vi "Kalman Filter Step.vi"(9 "Control Input":T2, 10 "Observations":T2, 11 "Kalman Filter In":T1) -> (3 "Kalman Filter Out":T1)   [LabVIEW 2020]
uses:
  ctl/Kalman Filter Instance.ctl
  <vilib>/Analysis/Matrix/Datatypes/RealMatrix.ctl
  ctl/Dynamical System Matrices.ctl
  <vilib>/Analysis/Matrix/NI_Matrix.lvlib
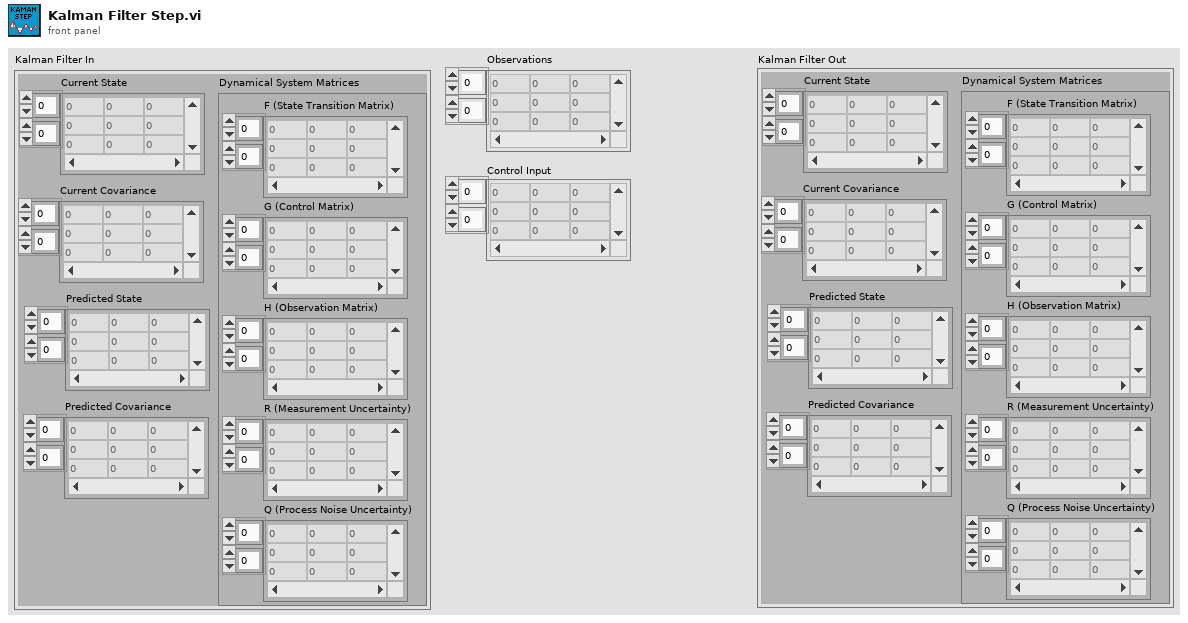
[diagram p1: front panel]
types:
  T1 = typedef "Kalman Filter Instance.ctl" = cluster{"Current State":T2, "Current Covariance":T2, "Predicted State":T2, "Predicted Covariance":T2, "Dynamical System Matrices":T3}
  T2 = typedef "NI_Matrix.lvlib/RealMatrix.ctl" = dbl[][]
  T3 = typedef "Dynamical System Matrices.ctl" = cluster{"F (State Transition Matrix)":T2, "G (Control Matrix)":T2, "H (Observation Matrix)":T2, "R (Measurement Uncertainty)":T2, "Q (Process Noise Uncertainty)":T2}
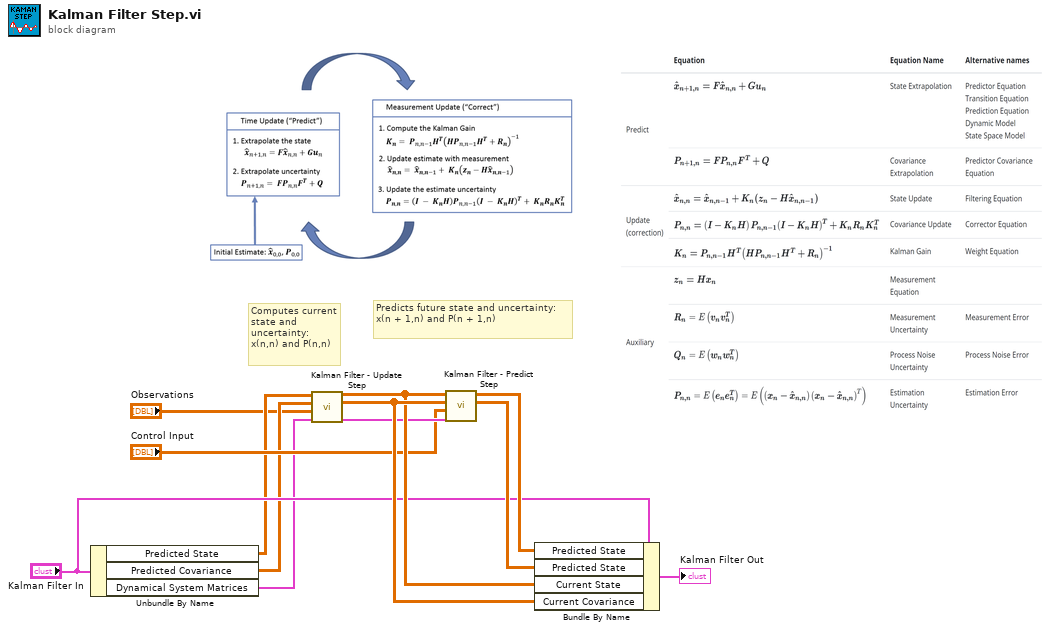
[diagram p0: block diagram]
diagram:
  # "Predicts future state and uncertainty: x(n + 1,n) and P(n + 1,n)"
  # "Computes current state and uncertainty: x(n,n) and P(n,n)"
  n1 = Unbundle By Name("Kalman Filter In") -> ("Predicted State"=w3:T2, "Predicted Covariance"=w4:T2, "Dynamical System Matrices"=w2:T3)
  n2 = call "Kalman Filter - Update Step.vi"("Dynamical System Matrices In"=w2, "Observations"="Observations", "Old Covariance"=w4, "Old State"=w3) -> ("Dynamical System Matrices Out"=w6:T3, "Updated Covariance"=w9:T2, "Updated State"=w8:T2)  [unwired: 5 in]
  n3 = call "Kalman Filter - Predict Step.vi"("Dynamical System Matrices In"=w6, "Control Input"="Control Input", "Initial Covariance"=w9, "Initial State"=w8) -> ("Predicted Covariance"=w11:T2, "Predicted State"=w10:T2)  [unwired: 5 in, 1 out]
  n4 = Bundle By Name(cluster="Kalman Filter In", "Predicted State"=w10, "Predicted State"=w11, "Current State"=w8, "Current Covariance"=w9) -> (→"Kalman Filter Out":T1)
